vi "Voltage Output Test.vi"(0 "DMM In":string="DMM", 5 "DMM Channel":i32, 7 "Power Supply In":string="PowerSupply", 9 "Line In":dbl, 11 "Error In":errorcluster) -> (4 "Output Voltage":dbl, 15 "Error Out":errorcluster)   [LabVIEW 2015]
doc: "Measures the output DC voltage when providing an input voltage from the battery pins."
uses:
  <instrlib>/Driver Simulation/DMM/Signal Types.ctl
  <instrlib>/Driver Simulation/Power Supply.lvlib
  <instrlib>/Driver Simulation/DMM.lvlib
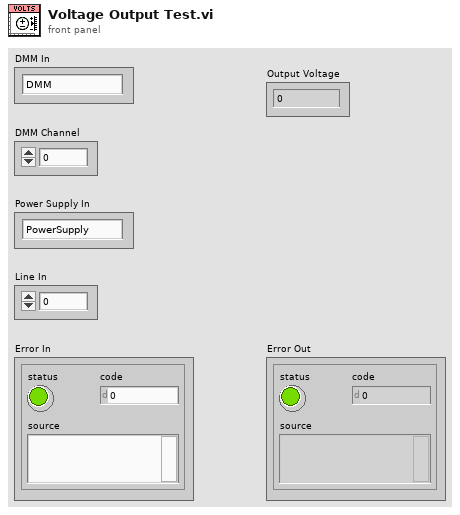
[diagram p1: front panel]
types:
  T1 = typedef "Driver Simulation.lvlib/DMM.lvlib/Signal Types.ctl" = enum16{"DC", "AC"}
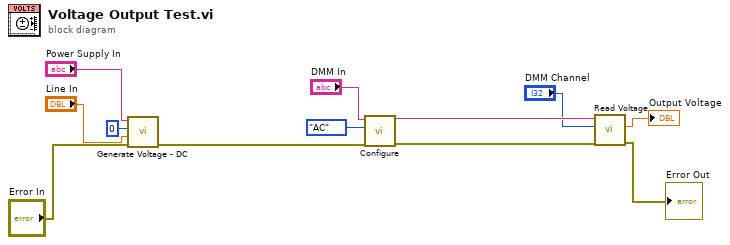
[diagram p0: block diagram]
diagram:
  n1 = call <instrlib>:"Generate Voltage - DC.vi"("error in (no error)"="Error In", "Output Voltage"="Line In", "Channel"=0, "Power Supply in"="Power Supply In") -> ("error out"=w10:errorcluster)  [unwired: 6 in, 1 out]
  n2 = call <instrlib>:"Configure.vi"("error in (no error)"=w10, "Signal Type"=Signal_Types."AC", "DMM in"="DMM In") -> ("error out"=w9:errorcluster, "DMM out"=w5:string)  [unwired: 7 in]
  n3 = call <instrlib>:"Read Voltage.vi"("error in (no error)"=w9, "Channel"="DMM Channel", "DMM in"=w5) -> ("error out"=→"Error Out":errorcluster, "Voltage"=→"Output Voltage":dbl)  [unwired: 6 in, 1 out]
